vi "Actor Core.vi"(8 "error in":errorcluster, 11 "ConcreteModel in":refnum<class "ConcreteModel.lvclass">) -> (0 "error out":errorcluster, 3 "Actor out":refnum<class "Actor.lvclass">)   [LabVIEW 2015, in "TopLevelApplication.lvlib" / "ConcreteModel.lvclass"]
doc: "(<B>Filename</B>: Actor Framework.lvlib:Actor.lvclass:Actor Core.vi)\n\nReceives messages to the actor, reacts to them, and initiates any error handling that may shut the actor down.\n\nDescendant classes may override this VI to append parallel tasks for the actor to complete while it handles messages. Overrides use the Call Parent Method node."
uses:
  ConcreteModel.lvclass
  <vilib>/ActorFramework/Actor/Actor.lvclass
  IModel/IModel/IModel.lvclass/IModel.ctl
  AbstractMessages/PreAddressedMsg/PreAddressedMsg.lvclass/PreAddressedMsg.ctl
  IMediator/IMediator Messages/Publish Msg/Publish Msg.lvclass/Publish Msg.ctl
  <vilib>/ActorFramework/Message Enqueuer/Message Enqueuer.lvclass/Message Enqueuer.ctl
  IMediator/IMediator Messages/Publish Msg/Send Publish.vi
  <vilib>/ActorFramework/Message Enqueuer/Enqueue.vi
  AbstractMessages/PreAddressedMsg/Read Return Address.vi
  <vilib>/ActorFramework/Message Priority Queue/Priority Enqueue.vi
  IModel/IModel/IModel.lvclass
panel:
  in  "Publish Period [ms]":u32=10
  in  "Stop Button":bool
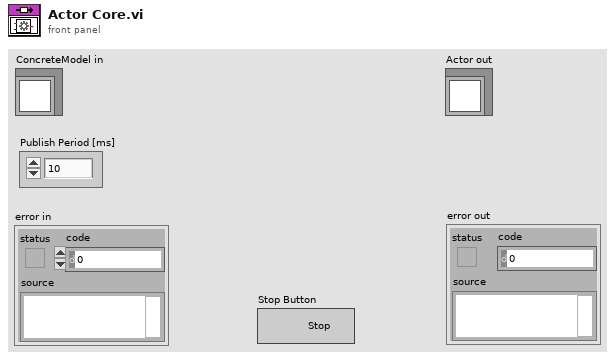
[diagram p1: front panel]
types:
  T1 = cluster{"seconds since 1Jan1904":timestamp, "number: 0 to 1":dbl}
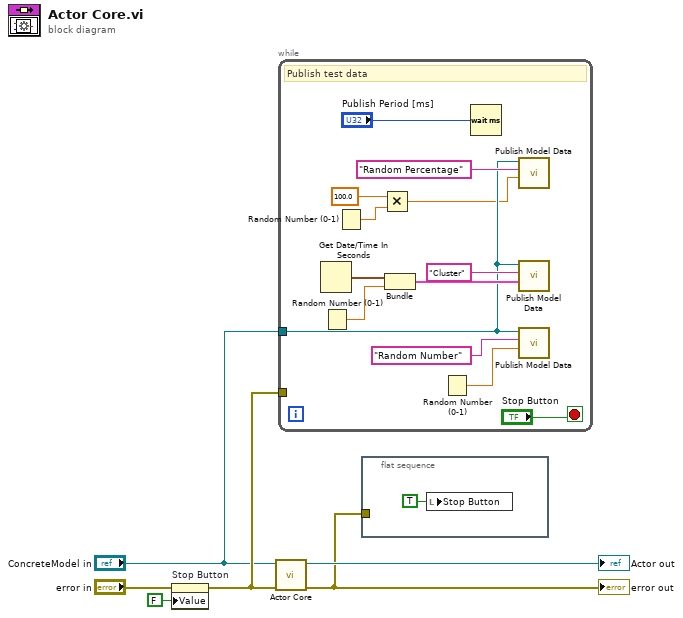
[diagram p0: block diagram]
diagram:
  n1 = property on="Stop Button" class="Bool (strict)"(error in="error in", "Value"=FALSE ("Stop Button")) -> (error out=w3:errorcluster)  [unwired: 1 in, 1 out]
  n2 = call-parent "Actor Core.vi"("error in"=w3, "Actor in"="ConcreteModel in") -> ("error out"=w1:errorcluster, "Actor out"=→"Actor out":refnum<class "Actor.lvclass">)  [unwired: 8 in]
  "error out" <- w1
  n3 = while {
    tunnel: w3 -> [_]
    tunnel: "ConcreteModel in" -> [w10]
    stop <- "Stop Button" stop-if-true
    # "Publish test data"
    n4 = Get Date/Time In Seconds() -> (seconds since 1Jan1904=w14:timestamp)
    n5 = Random Number (0-1)() -> (number: 0 to 1=w15:dbl)
    n6 = Random Number (0-1)() -> (number: 0 to 1=w9:dbl)
    n7 = Multiply(x=100.0, y=w9) -> (x*y=w7:dbl)
    n8 = Bundle("seconds since 1Jan1904"=w14, "number: 0 to 1"=w15) -> (w13:T1)  [unwired: 1 in]
    n9 = Random Number (0-1)() -> (number: 0 to 1=w17:dbl)
    n10 = Wait (ms)(milliseconds to wait="Publish Period [ms]") -> ()  [unwired: 1 out]
    n11 = call "Publish Model Data.vi"("Data to Publish"=w7, "Topic Name"="Random Percentage", "IModel in"=w10) -> ()  [unwired: 7 in, 2 out]
    n12 = call "Publish Model Data.vi"("Data to Publish"=w13, "Topic Name"="Cluster", "IModel in"=w10) -> ()  [unwired: 7 in, 2 out]
    n13 = call "Publish Model Data.vi"("Data to Publish"=w17, "Topic Name"="Random Number", "IModel in"=w10) -> ()  [unwired: 7 in, 2 out]
  }
  n14 = flat-sequence {
    tunnel: w1 -> [_]
    frame #0 {
      n15 = local write "Stop Button"(TRUE ("Stop Button")) -> ()
    }
  }
